vi "Read Source.vi"(8 "Error In":errorcluster, 11 "Node In":refnum<class "Node.lvclass">) -> (0 "Error Out":errorcluster, 2 "Source":string, 3 "Node Out":refnum<class "Node.lvclass">)   [LabVIEW 2018, in "Toolkit.lvlib" / "Nodes.lvlib" / "Node.lvclass"]
doc: "Gets the original, raw text from the Mustache template that yielded the node during the parsing process.\n\n<B>Node In/Out</B> - Represents a node in the Abstract Syntax Tree (AST) of a parsed Mustache template.\n\n<B>Source</B> - The original, raw text from the Mustache template."
uses:
  Node.lvclass
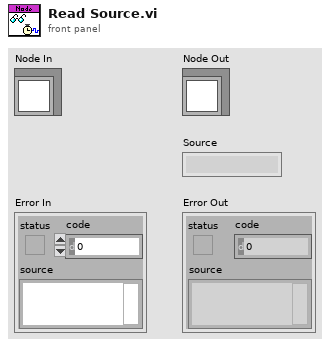
[diagram p1: front panel]
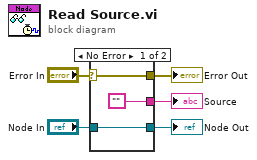
[diagram p0: block diagram]
diagram:
  n1 = case shown="No Error" "Error In" {
    selector: "Error In" -> [w8 w9]
    tunnel: [w8 w9] -> w4
    tunnel: [w7 w10] -> w2
    tunnel: "Node In" -> [w7 w10]
    tunnel: ["" _] -> w1
    frame No Error {
    }
    frame Error {
    }
  }
  "Error Out" <- w4
  "Node Out" <- w2
  "Source" <- w1
